vi "SetFrontEndDef.vi"(8 "error in (no error)":errorcluster, 11 "FE_DEF":T1) -> (0 "error out":errorcluster)   [LabVIEW 2011]
uses:
  Front End Definition.ctl
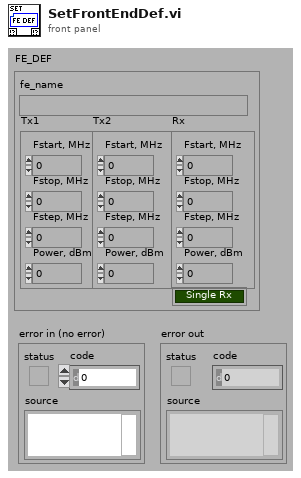
[diagram p1: front panel]
types:
  T1 = typedef "Front End Definition.ctl" = cluster{"fe_name":string, "Tx1":cluster{"Fstart, MHz":dbl, "Fstop, MHz":dbl, "Fstep, MHz":dbl, "Power, dBm":dbl}, "Tx2":cluster{"Fstart, MHz":dbl, "Fstop, MHz":dbl, "Fstep, MHz":dbl, "Power, dBm":dbl}, "Rx":cluster{"Fstart, MHz":dbl, "Fstop, MHz":dbl, "Fstep, MHz":dbl, "Power, dBm":dbl}, "BothSides":bool}
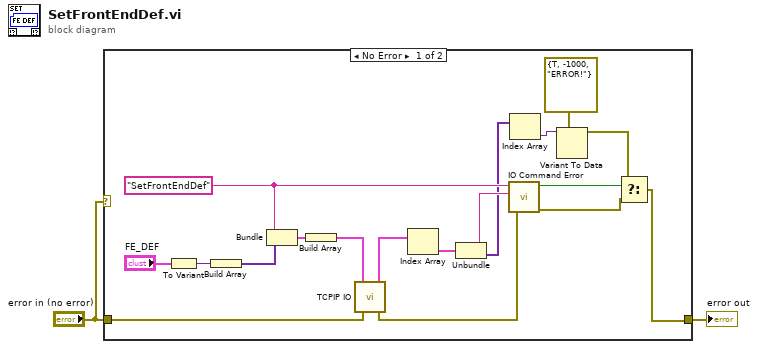
[diagram p0: block diagram]
diagram:
  n1 = case shown="No Error" "error in (no error)" {
    tunnel: "error in (no error)" -> [w18 w21]
    tunnel: [w3 w21] -> w2
    frame No Error {
      w16 = "SetFrontEndDef"
      n2 = To Variant(anything="FE_DEF") -> (Variant=w20:variant)
      n3 = Build Array(w20) -> (w19:variant[])
      n4 = Bundle(w16, w19) -> (w17:cluster{string, variant[]})  [unwired: 1 out]
      n5 = Build Array(w17) -> (w14:cluster{string, variant[]}[])
      n6 = call "TCPIP IO.vi"("error in (no error)"=w18, "Commands"=w14) -> ("error out"=w15:errorcluster, "Responses"=w13:cluster{string, variant[]}[])  [unwired: 1 in, 3 out]
      n7 = Index Array(array=w13) -> (element=w12:cluster{string, variant[]})  [unwired: 1 in]
      n8 = Unbundle(w12) -> (w11:string, w5:variant[])
      n9 = call "IO Command Error.vi"("error in (no error)"=w15, "Command Returned (\"\")"=w11, "Command Sent (\"\")"=w16) -> ("error out"=w4:errorcluster, "HW ERR?"=w6:bool)  [unwired: 3 out]
      n10 = Index Array(array=w5) -> (element=w9:variant)  [unwired: 1 in]
      n11 = Variant To Data(type=errorcluster {"status"=TRUE, "code"=-1000, "source"="ERROR!"} ("error out"), Variant=w9) -> (data=w7:errorcluster)  [unwired: 1 in, 1 out]
      n12 = Select(t=w7, s=w6, f=w4) -> (s? t:f=w3:errorcluster)
    }
    frame Error {
    }
  }
  "error out" <- w2
